vi "Get cmd info from step name.vi"(10 "Select Command":string, 11 "Command Library Data":string[][](array[string])) -> (1 "Expected response size (bytes":i32, 2 "cmd opcode (string)":string, 3 "cmd name":string)   [LabVIEW 2020]
uses:
  d77d80d3-7f66-4ff4-94d1-612bb61cf61d.vi
  <vilib>/Comparison/Equal/Equal Functor/Equal Functor.lvclass
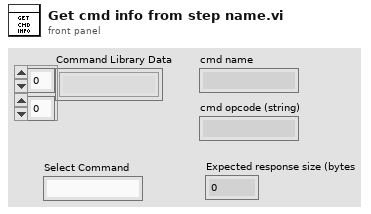
[diagram p1: front panel]
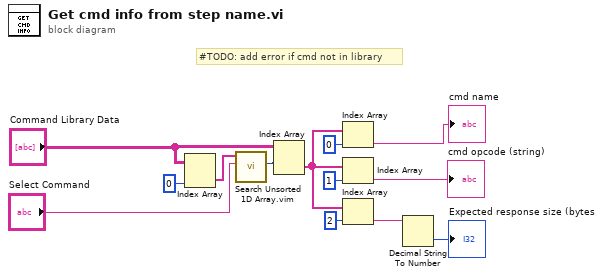
[diagram p0: block diagram]
diagram:
  # "#TODO: add error if cmd not in library"
  n1 = Index Array(array="Command Library Data", index (col)=0 ("disabled index (col)")) -> (element=w5:string[])  [unwired: 1 in]
  n2 = call "Search Unsorted 1D Array.vim"("element"="Select Command", "unsorted 1D array"=w5) -> ("index of element"=w7:i32)  [unwired: 9 in]
  n3 = Index Array(array="Command Library Data", index (row)=w7) -> (element=w2:string[])  [unwired: 1 in]
  n4 = Index Array(array=w2, index=0) -> (element=→"cmd name":string)
  n5 = Index Array(array=w2, index=1) -> (element=→"cmd opcode (string)":string)
  n6 = Index Array(array=w2, index=2) -> (element=w12:string)
  n7 = Decimal String To Number(string=w12) -> (number=→"Expected response size (bytes":i32)  [unwired: 2 in, 1 out]
